vi "Load.Signals.Convert.1_0_1 to 3_0_0.vi"(11 "Signals":T1(array[cluster])) -> (3 "Signals":T2[](array[typedef]) {"Signals"."Byte Order" items=["Little Endian", "Big Endian"]; "Signals"."Data Type" items=["Signed", "Unsigned", "IEEE Float"]})   [LabVIEW 2015, in "Diagnostics Addon System Explorer.lvlib"]
uses:
  Diagnostics Addon System Explorer.lvlib
  Types/Frame.Export.ctl
  Shared/Types/Signal.ctl
  Shared/Diagnostics Addon Shared.lvlib
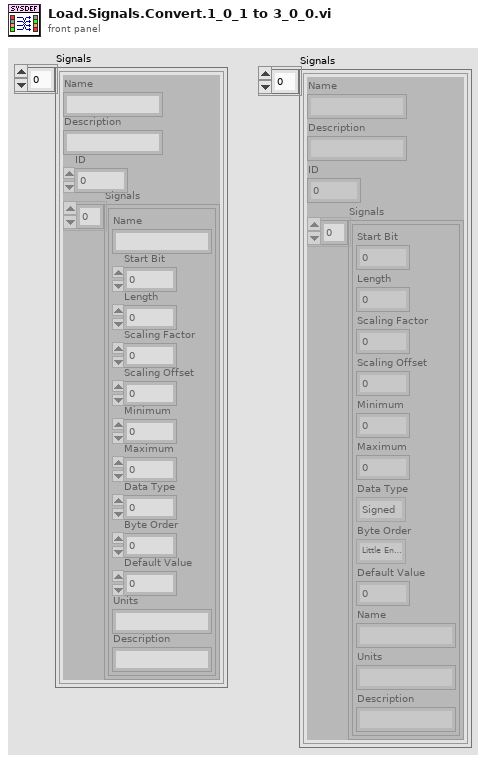
[diagram p1: front panel]
types:
  T1 = cluster{"Name":string, "Description":string, "ID":u16, "Signals":cluster{"Name":string, "Start Bit":u8, "Length":u8, "Scaling Factor":dbl, "Scaling Offset":dbl, "Minimum":dbl, "Maximum":dbl, "Data Type":u32, "Byte Order":u32, "Default Value":dbl, "Units":string, "Description":string}[]}[]
  T2 = typedef "Diagnostics Addon System Explorer.lvlib/Frame.Export.ctl" = cluster{"Name":string, "Description":string, "ID":u32, "Signals":T3[]}
  T3 = typedef "Diagnostics Addon Shared.lvlib/Signal.ctl" = cluster{"Start Bit":u32, "Length":u32, "Scaling Factor":dbl, "Scaling Offset":dbl, "Minimum":dbl, "Maximum":dbl, "Data Type":u32, "Byte Order":u32, "Default Value":dbl, "Name":string, "Units":string, "Description":string}
  T4 = cluster{"Name":string, "Start Bit":u8, "Length":u8, "Scaling Factor":dbl, "Scaling Offset":dbl, "Minimum":dbl, "Maximum":dbl, "Data Type":u32, "Byte Order":u32, "Default Value":dbl, "Units":string, "Description":string}[]
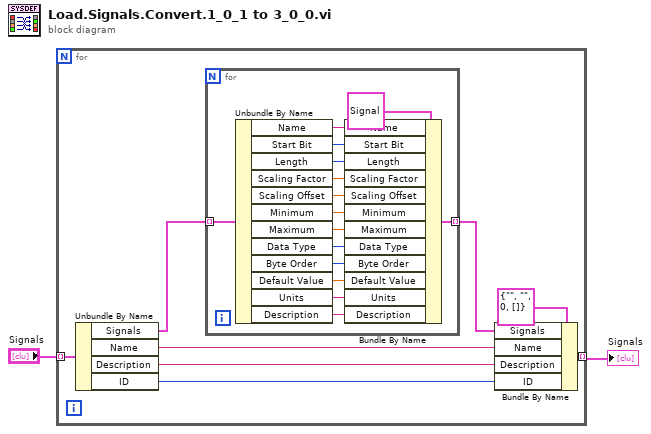
[diagram p0: block diagram]
diagram:
  n1 = for {
    tunnel: "Signals" -> [w9] mode=indexing
    tunnel: [w6] -> w2 mode=indexing
    n2 = Unbundle By Name(w9) -> ("Signals"=w10:T4, "Name"=w5:string, "Description"=w4:string, "ID"=w3:u16)
    n3 = for {
      tunnel: w10 -> [w12] mode=indexing
      tunnel: [w11] -> w8 mode=indexing
      n4 = Unbundle By Name(w12) -> ("Name"=w14:string, "Start Bit"=w15:u8, "Length"=w16:u8, "Scaling Factor"=w17:dbl, "Scaling Offset"=w18:dbl, "Minimum"=w19:dbl, "Maximum"=w20:dbl, "Data Type"=w21:u32, "Byte Order"=w22:u32, "Default Value"=w23:dbl, "Units"=w24:string, "Description"=w25:string)
      n5 = Bundle By Name(cluster=T3 {"Start Bit"=0, "Length"=0, "Scaling Factor"=0.0, "Scaling Offset"=0.0, "Minimum"=0.0, "Maximum"=0.0, "Data Type"=0, "Byte Order"=0, "Default Value"=0.0, "Name"="", "Units"="", "Description"=""} ("Signal Parameters"), "Name"=w14, "Start Bit"=w15, "Length"=w16, "Scaling Factor"=w17, "Scaling Offset"=w18, "Minimum"=w19, "Maximum"=w20, "Data Type"=w21, "Byte Order"=w22, "Default Value"=w23, "Units"=w24, "Description"=w25) -> (w11:T3)
    }
    n6 = Bundle By Name(cluster=T2 {"Name"="", "Description"="", "ID"=0, "Signals"=[]} ("DIDPID"), "Signals"=w8, "Name"=w5, "Description"=w4, "ID"=w3) -> (w6:T2)
  }
  "Signals" <- w2
